vi "Parse Input.vi"(11 "Input":string) -> (3 "Puzzle":T1)   [LabVIEW 2020]
uses:
  Puzzle.ctl
  Dot.ctl
  Fold.ctl
  Axis.ctl
  <vilib>/regexp/Match Regular Expression.xnode
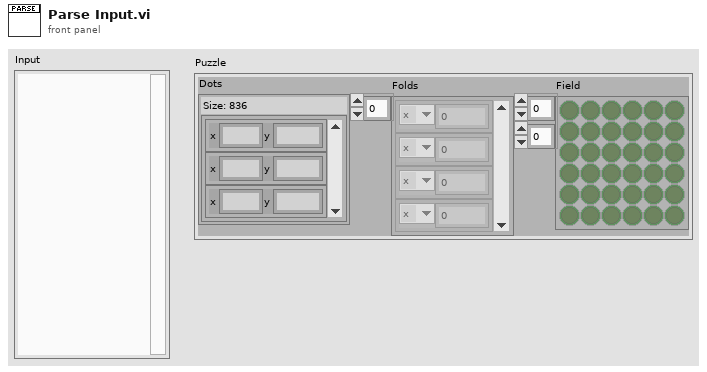
[diagram p1: front panel]
types:
  T1 = typedef "Puzzle.ctl" = cluster{"Dots":set{T2}, "Folds":T3[], "Field":bool[][]}
  T2 = typedef "Dot.ctl" = cluster{"x":i32, "y":i32}
  T3 = typedef "Fold.ctl" = cluster{"Axis":T4, "Value":i32}
  T4 = typedef "Axis.ctl" = enum16{"x", "y"}
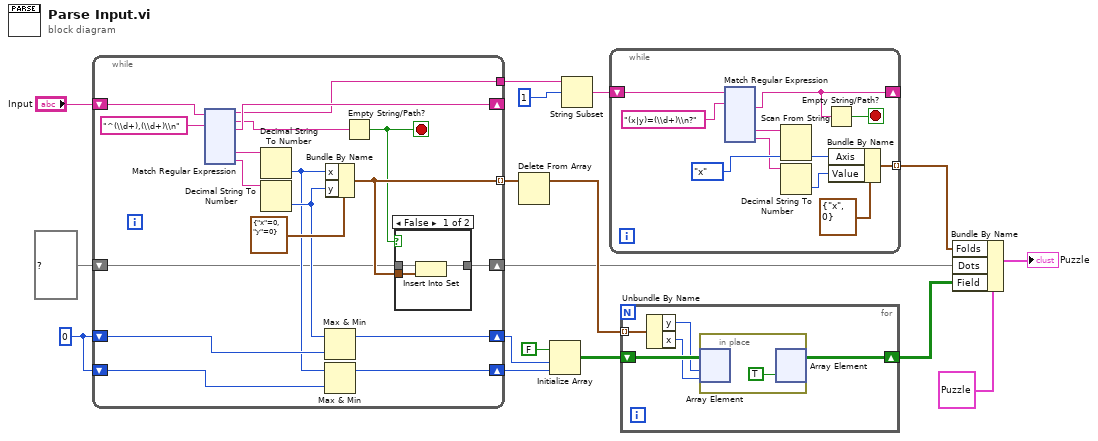
[diagram p0: block diagram]
diagram:
  w10 = 0
  n1 = while {
    shift-right: [w33] -> _
    shift-left: "Input" -> [w35]
    tunnel: [w32] -> w16
    tunnel: [w20] -> w5 mode=indexing
    shift-right: [w27] -> w8
    shift-left: w10 -> [w26]
    shift-right: [w25] -> w9
    shift-left: w10 -> [w24]
    shift-right: [w21] -> w1
    shift-left: set{T2} {} ("Dots") -> [w19]
    stop <- w18 stop-if-true
    n2 = xnode "Match Regular Expression"("input string"=w35, "regular expression"="^(\\d+),(\\d+)\\n") -> ("before match"=w32:string, "whole match"=w31:string, "after match"=w33:string, "submatch 1"=w30:string, "submatch 2"=w29:string)  [unwired: 4 in, 2 out]
    n3 = Decimal String To Number(string=w30) -> (number=w22:i32)  [unwired: 2 in, 1 out]
    n4 = Decimal String To Number(string=w29) -> (number=w23:i32)  [unwired: 2 in, 1 out]
    n5 = Max & Min(x=w23, y=w26) -> (max(x,y)=w27:i32)  [unwired: 1 out]
    n6 = Max & Min(x=w22, y=w24) -> (max(x,y)=w25:i32)  [unwired: 1 out]
    n7 = Bundle By Name(cluster=T2 {"x"=0, "y"=0} ("Dot"), "x"=w22, "y"=w23) -> (w20:T2)
    n8 = Empty String/Path?(string/path=w31) -> (empty?=w18:bool)
    n9 = case shown="False" w18 {
      tunnel: [w38 w39] -> w21
      tunnel: w20 -> [w37 _]
      tunnel: w19 -> [w36 w39]
      frame False {
        n10 = Insert Into Set(10:w37, 11:w36) -> (3:w38:set{T2})  [unwired: 1 out]
      }
      frame True {
      }
    }
  }
  n11 = Delete From Array(array=w5) -> (array with subset deleted=w3:T2[])  [unwired: 2 in, 1 out]
  n12 = Initialize Array(FALSE, w8, w9) -> (w6:bool[][])
  n13 = String Subset(string=w16, offset (0)=1) -> (substring=w14:string)  [unwired: 1 in]
  n14 = while {
    shift-right: [w158] -> _
    shift-left: w14 -> [w167]
    tunnel: [w159] -> w12 mode=indexing
    stop <- w157 stop-if-true
    n15 = xnode "Match Regular Expression"("input string"=w167, "regular expression"="(x|y)=(\\d+)\\n?") -> ("after match"=w158:string, "submatch 1"=w165:string, "submatch 2"=w161:string)  [unwired: 4 in, 4 out]
    n16 = Scan From String(input string=w165, default 1=Axis."x" ("Axis")) -> (output 1=w162:T4)  [unwired: 3 in, 3 out]
    n17 = Decimal String To Number(string=w161) -> (number=w160:i32)  [unwired: 2 in, 1 out]
    n18 = Empty String/Path?(string/path=w158) -> (empty?=w157:bool)
    n19 = Bundle By Name(cluster=T3 {"Axis"=enum."x", "Value"=0} ("Fold"), "Axis"=w162, "Value"=w160) -> (w159:T3)
  }
  n20 = for {
    shift-right: [w285] -> w4
    shift-left: w6 -> [w288]
    tunnel: w3 -> [w289] mode=indexing
    n21 = Unbundle By Name(w289) -> ("y"=w286:i32, "x"=w287:i32)
    n22 = in-place {
      n23 = in-place-array #1(w288, w286, w287) -> ()  [unwired: 1 out]
      n24 = in-place-array #1(TRUE) -> (w285:bool[][])  [unwired: 2 out]
    }
  }
  n25 = Bundle By Name(cluster=T1 {"Dots"={}, "Folds"=[], "Field"=[]} ("Puzzle"), "Folds"=w12, "Dots"=w1, "Field"=w4) -> (→"Puzzle":T1)
